vi "Manual Control.vi"() -> ()   [LabVIEW 2013]
panel:
  out "thin set":i32
  out "thick set":i32
  in  "Step Size":i32=25
  in  "Stop Button":bool
  # "Use the arrow keys on the keybard to control the etalons\nSelect speeds from 10 to 100 by the top row number keys"
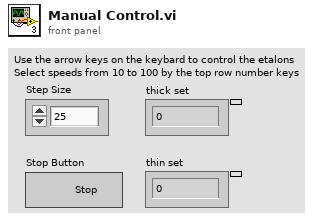
[diagram p1: front panel]
types:
  T1 = typedef "eventvkey.ctl" = enum16{"ASCII", "Enter", "Return", "Shift", "Ctrl", "Alt", "Cmd", "Opt", "Caps", "NumLock", "Clear", "Break", "Up", "Down", "Left", "Right", "Insert", "Delete", "Home", "End", "PageUp", "PageDown", "Escape", "Help", "Pause", "ScrollLock", "F1", "F2", "F3", "F4", "F5", "F6", "F7", "F8", "F9", "F10", "F11", "F12", "F13", "F14", "F15", "F16", "F17", "F18", "F19", "F20", "F21", "F22", "F23", "F24", "Play", "VolumeUp", "VolumeDown", "Mute", "Two Byte Char"}
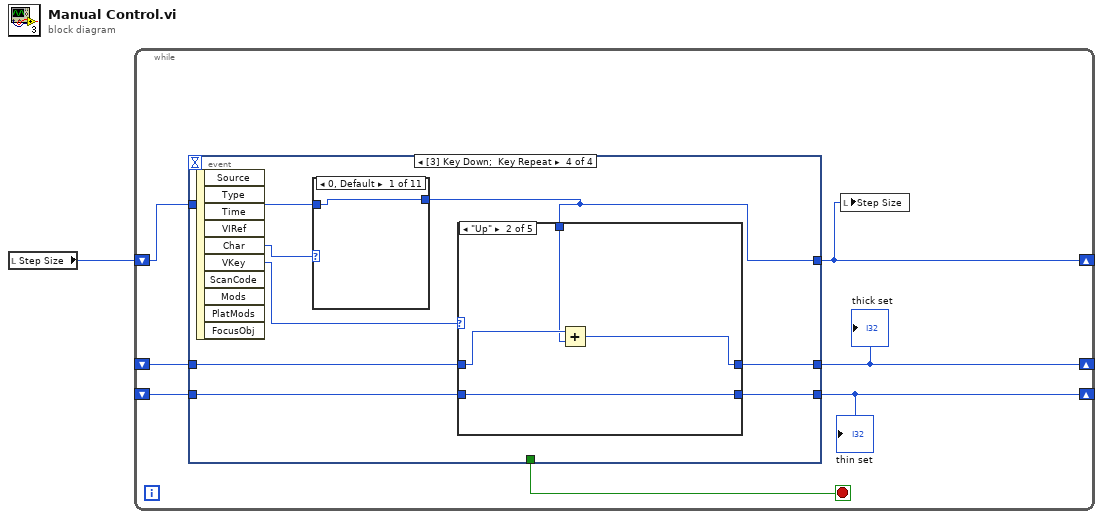
[diagram p0: block diagram]
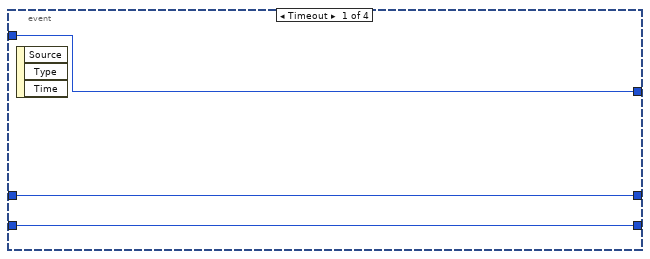
[diagram p2: hidden frame]
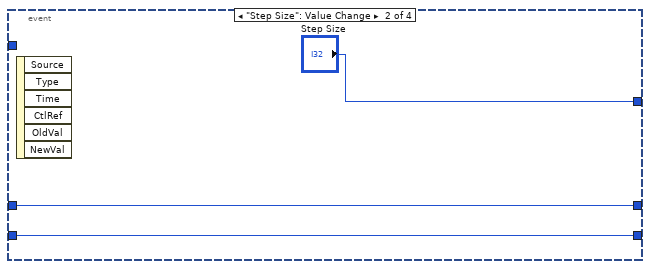
[diagram p3: hidden frame]
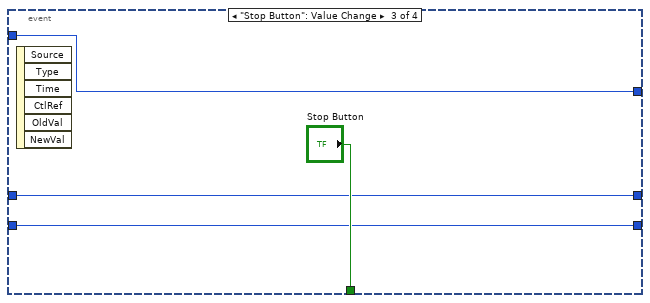
[diagram p4: hidden frame]
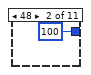
[diagram p5: hidden frame]
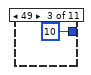
[diagram p6: hidden frame]
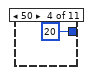
[diagram p7: hidden frame]
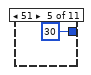
[diagram p8: hidden frame]
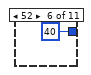
[diagram p9: hidden frame]
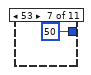
[diagram p10: hidden frame]
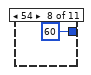
[diagram p11: hidden frame]
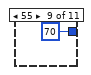
[diagram p12: hidden frame]
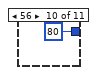
[diagram p13: hidden frame]
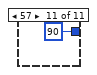
[diagram p14: hidden frame]
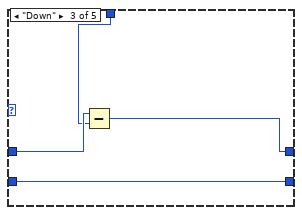
[diagram p16: hidden frame]
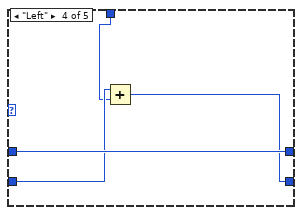
[diagram p17: hidden frame]
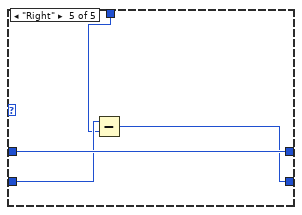
[diagram p18: hidden frame]
diagram:
  n1 = local read "Step Size"() -> (w1:i32)
  n2 = while {
    shift-right: [w5] -> _
    shift-left: _ -> [w7]
    shift-right: [w3] -> _
    shift-left: _ -> [w6]
    shift-right: [w2] -> _
    shift-left: w1 -> [w4]
    stop <- w8 stop-if-true
    n3 = event shown="[3] Key Down;  Key Repeat" {
      selector: _ -> [_ _ _ _]
      dyn-events: _ -> [_ _ _ _]
      timeout: _ -> [_ _ _ _]
      tunnel: [_ _ "Stop Button" _] -> w8
      tunnel: w7 -> [w11 w14 w16 w25]
      tunnel: w6 -> [w10 w13 w17 w24]
      tunnel: [w11 w14 w16 w23] -> w5
      tunnel: [w10 w13 w17 w22] -> w3
      tunnel: [w9 "Step Size" w15 w20] -> w2
      tunnel: w4 -> [w9 _ w15 w19]
      event Timeout {
        n4 = event-data() -> ()  [unwired: 1 in, 3 out]
      }
      event "Step Size": Value Change {
        n5 = event-data() -> ()  [unwired: 1 in, 6 out]
      }
      event "Stop Button": Value Change {
        n6 = event-data() -> ()  [unwired: 1 in, 6 out]
      }
      event Key Down; Key Repeat {
        n7 = event-data() -> ("Char"=w21:i16, "VKey"=w26:T1)  [unwired: 1 in, 8 out]
        n8 = case shown="0, Default" w21 {
          tunnel: [w27 100 ("Step Size") 10 ("Step Size") 20 ("Step Size") 30 ("Step Size") 40 ("Step Size") 50 ("Step Size") 60 ("Step Size") 70 ("Step Size") 80 ("Step Size") 90 ("Step Size")] -> w20
          tunnel: w19 -> [w27 _ _ _ _ _ _ _ _ _ _]
          frame 0, Default {
          }
          frame 48 {
          }
          frame 49 {
          }
          frame 50 {
          }
          frame 51 {
          }
          frame 52 {
          }
          frame 53 {
          }
          frame 54 {
          }
          frame 55 {
          }
          frame 56 {
          }
          frame 57 {
          }
        }
        n9 = case shown="\"Up\"" w26 {
          tunnel: w25 -> [w39 w41 w45 w51 w55]
          tunnel: w24 -> [w38 w43 w47 w50 w54]
          tunnel: [w39 w42 w46 w51 w55] -> w23
          tunnel: [w38 w43 w47 w48 w52] -> w22
          tunnel: w20 -> [_ w40 w44 w49 w53]
          frame "ASCII", Default {
          }
          frame "Up" {
            n10 = Add(x=w41, y=w40) -> (x+y=w42:i32)
          }
          frame "Down" {
            n11 = Subtract(x=w45, y=w44) -> (x-y=w46:i32)
          }
          frame "Left" {
            n12 = Add(x=w50, y=w49) -> (x+y=w48:i32)
          }
          frame "Right" {
            n13 = Subtract(x=w54, y=w53) -> (x-y=w52:i32)
          }
        }
      }
    }
    "thick set" <- w5
    "thin set" <- w3
    n14 = local write "Step Size"(w2) -> ()
  }
